vi "Benchmark Creation.vi"(8 "error in (no error)":errorcluster, 11 "CIFCorePlugin in":refnum<class "CIFCorePlugin.lvclass">) -> (0 "error out":errorcluster, 3 "CIFCorePlugin out":refnum<class "CIFCorePlugin.lvclass">)   [LabVIEW 2021, in "CIFCorePlugin.lvclass"]
uses:
  CIFCorePlugin.lvclass
  CIFCorePlugin.lvclass/CIFCorePlugin.ctl
  <vilib>/CIF Foundation/CIF Utilities/Statistics/I64/Stats_I64_CIF_U.lvclass/Stats_I64_CIF_U.ctl
  <vilib>/CIF Foundation/CIF Utilities/Time/System Time/LabVIEW Time to TAI Time.vi
  <vilib>/CIF Foundation/CIF Utilities/Statistics/I64/Stats_I64_CIF_U.lvclass
  <vilib>/CIF Foundation/CIF Utilities/Time/Time_CIF_U.lvlib
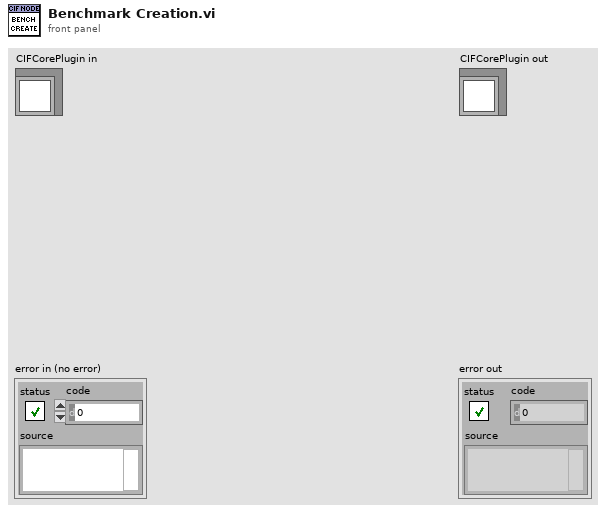
[diagram p1: front panel]
types:
  T1 = typedef "CIFCorePlugin.lvclass/Benchmarks.ctl" = cluster{"Period":refnum<class "Stats_I64_CIF_U.lvclass">, "Wake Error":refnum<class "Stats_I64_CIF_U.lvclass">, "Execute":refnum<class "Stats_I64_CIF_U.lvclass">, "Housekeep":refnum<class "Stats_I64_CIF_U.lvclass">, "Idle":refnum<class "Stats_I64_CIF_U.lvclass">, "Cleanup":refnum<class "Stats_I64_CIF_U.lvclass">, "FIFO T0":refnum<class "Stats_I64_CIF_U.lvclass">, "FIFO Prev PU":refnum<class "Stats_I64_CIF_U.lvclass">, "Output Error":refnum<class "Stats_I64_CIF_U.lvclass">, "Custom 1":refnum<class "Stats_I64_CIF_U.lvclass">, "Custom 2":refnum<class "Stats_I64_CIF_U.lvclass">}
  T2 = cluster{"[0]":refnum<class "Stats_I64_CIF_U.lvclass">, "[1]":refnum<class "Stats_I64_CIF_U.lvclass">, "[2]":refnum<class "Stats_I64_CIF_U.lvclass">, "[3]":refnum<class "Stats_I64_CIF_U.lvclass">, "[4]":refnum<class "Stats_I64_CIF_U.lvclass">, "[5]":refnum<class "Stats_I64_CIF_U.lvclass">, "[6]":refnum<class "Stats_I64_CIF_U.lvclass">, "[7]":refnum<class "Stats_I64_CIF_U.lvclass">, "[8]":refnum<class "Stats_I64_CIF_U.lvclass">, "[9]":refnum<class "Stats_I64_CIF_U.lvclass">, "[10]":refnum<class "Stats_I64_CIF_U.lvclass">}
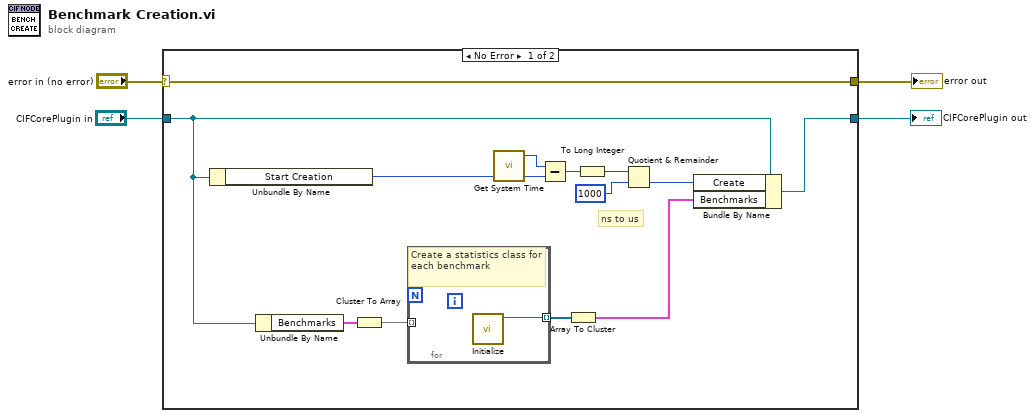
[diagram p0: block diagram]
diagram:
  n1 = case shown="No Error" "error in (no error)" {
    selector: "error in (no error)" -> [w10 w20]
    tunnel: [w10 w20] -> w2
    tunnel: [w17 w19] -> w1
    tunnel: "CIFCorePlugin in" -> [w9 w19]
    frame No Error {
      # "ns to us"
      n2 = Unbundle By Name(w9) -> ("Start Creation"=w16:i64)
      n3 = Unbundle By Name(w9) -> ("Benchmarks"=w8:T1)
      n4 = Cluster To Array(cluster=w8) -> (array=w6:refnum<class "Stats_I64_CIF_U.lvclass">[])
      n5 = for {
        tunnel: [w18] -> w5 mode=indexing
        tunnel: w6 -> [_] mode=indexing
        # "Create a statistics class for each benchmark"
        n6 = call <vilib>:"Initialize.vi"() -> ("Stats_I64_CIF_U out"=w18:refnum<class "Stats_I64_CIF_U.lvclass">)  [unwired: 10 in, 1 out]
      }
      n7 = call <vilib>:"Get System Time.vi"() -> ("Time (ns)"=w15:i64)  [unwired: 5 in]
      n8 = Subtract(x=w15, y=w16) -> (x-y=w13:i64)
      n9 = Array To Cluster(array=w5) -> (cluster=w7:T2)
      n10 = To Long Integer(number=w13) -> (32bit integer=w12:i32)
      n11 = Quotient & Remainder(x=w12, y=1000) -> (floor(x/y)=w11:i32)  [unwired: 1 out]
      n12 = Bundle By Name(cluster=w9, "Create"=w11, "Benchmarks"=w7) -> (w17:refnum<class "CIFCorePlugin.lvclass">)
    }
    frame Error {
    }
  }
  "error out" <- w2
  "CIFCorePlugin out" <- w1
